vi "ButtonExample.vi"() -> ()   [LabVIEW 2017]
panel:
  in  "stop":bool
  out "Boolean 2":bool
  in  "Boolean":bool
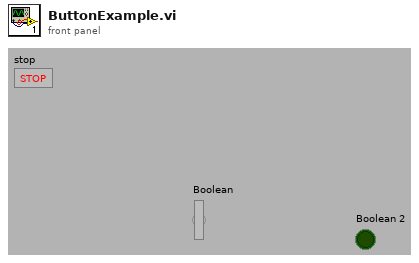
[diagram p1: front panel]
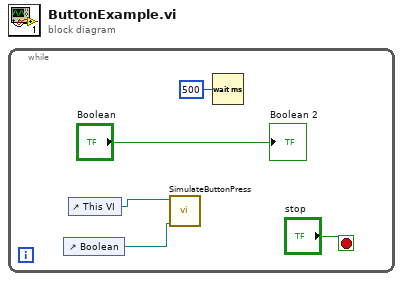
[diagram p0: block diagram]
diagram:
  n1 = while {
    stop <- "stop" stop-if-true
    n2 = control-ref of="Boolean"() -> (w2:refnum<vi>)
    n3 = control-ref of="This VI"() -> (w3:refnum<vi>)
    n4 = call "SimulateButtonPress.vi"("Reference to Button"=w2, "VI Reference"=w3) -> ()  [unwired: 10 in]
    n5 = Wait (ms)(milliseconds to wait=u32 500) -> ()  [unwired: 1 out]
    "Boolean 2" <- "Boolean"
  }
